vi "All Stream ID Sorted Transfers.vi"(1 "transfer groups":T1[](array[typedef])) -> (0 "stream-sorted transfers":T3[](array[typedef]))   [LabVIEW 2017, in "PXImc.lvlib" / "PXImc Transceiver.lvclass"]
uses:
  PXImc Transceiver.lvclass
  PXImc Transfer Data.ctl
  PXImc Group Data.ctl
  Builds/Data Sharing Framework/Current/Core/DSF Core.lvlibp/Typedefs/DSF Direction.ctl
  Builds/Data Sharing Framework/Current/Core/DSF Core.lvlibp
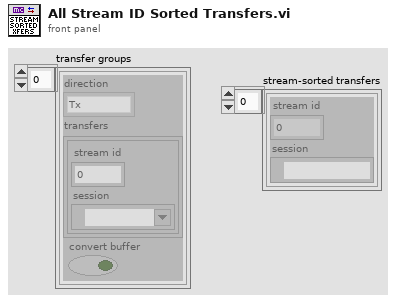
[diagram p1: front panel]
types:
  T1 = typedef "PXImc.lvlib/PXImc Transceiver.lvclass/PXImc Group Data.ctl" = cluster{"direction":T2, "transfers":T3[], "convert buffer":bool}
  T2 = typedef "DSF Core.lvlibp/DSF Direction.ctl" = enum8{"Tx", "Rx"}
  T3 = typedef "PXImc.lvlib/PXImc Transceiver.lvclass/PXImc Transfer Data.ctl" = cluster{"stream id":u16, "session":refnum<k21>}
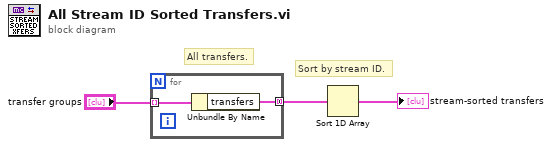
[diagram p0: block diagram]
diagram:
  # "All transfers."
  # "Sort by stream ID."
  n1 = for {
    tunnel: "transfer groups" -> [w5] mode=indexing
    tunnel: [w4] -> w2 mode=concatenating
    n2 = Unbundle By Name(w5) -> ("transfers"=w4:T3[])
  }
  n3 = Sort 1D Array(array=w2) -> (sorted array=→"stream-sorted transfers":T3[])
